vi "NewGame.vi"(7 "GPongType (ChildObject)":refnum<class "GPong.lvclass">, 8 "error in (no error)":errorcluster, 11 "FPGA_ref":T1) -> (0 "error out":errorcluster, 3 "GPong out":refnum<class "GPong.lvclass">)   [LabVIEW 2019, in "RT_Game.lvlib" / "GPong.lvclass"]
uses:
  GPong.lvclass
  C:/Users/FreshBob/Dropbox/VIs/myRIO_GameConsole/RT/RT_Game/Game/Game.lvclass
  FPGA_Interface.ctl
  Game/Game.lvclass/Game.ctl
  GameObject/GameObject.lvclass/GameObject.ctl
  Game/Read Sprite3.vi
  GameObject/Write MinSpeed.vi
  GameObject/Write MaxSpeed.vi
  GameObject/Write MaxSpeedX.vi
  GameObject/Write Damping.vi
  GameObject/Write Gravity.vi
  Game/Write Sprite3.vi
  RT_Sprite/RT_Sprite.lvclass
  C:/Users/FreshBob/Dropbox/VIs/myRIO_GameConsole/RT/RT_Game/GameObject/GameObject.lvclass
  Pong/Pong.lvclass
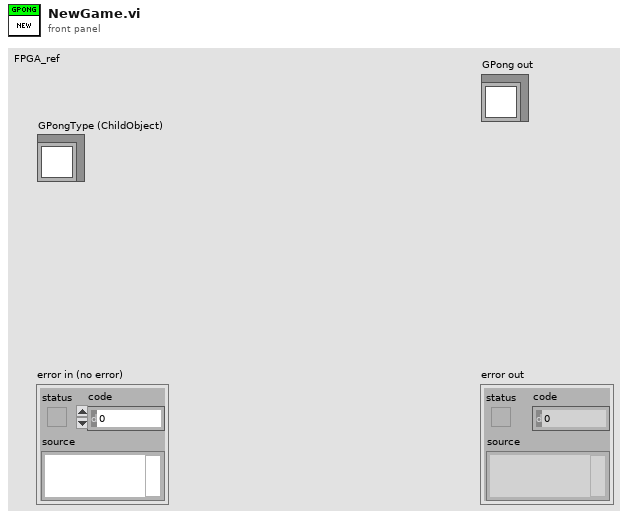
[diagram p1: front panel]
types:
  T1 = typedef "FPGA_Interface.ctl" = refnum<k20>
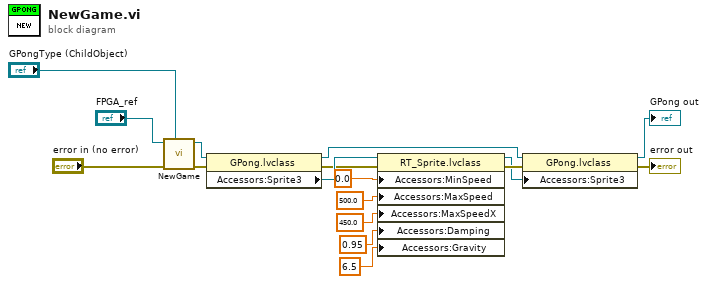
[diagram p0: block diagram]
diagram:
  n1 = call-parent "NewGame.vi"("PongType (ChildObject)"="GPongType (ChildObject)", "error in (no error)"="error in (no error)", "FPGA_ref"="FPGA_ref") -> ("error out"=w17:errorcluster, "Pong out"=w8:refnum<class "GPong.lvclass">)  [unwired: 7 in]
  n2 = property class="GPong.lvclass"(reference=w8, error in=w17) -> (reference out=w3:refnum<class "GPong.lvclass">, error out=w6:errorcluster, "Accessors:Sprite3"=w7:refnum<class "RT_Sprite.lvclass">)
  n3 = property class="RT_Sprite.lvclass"(reference=w7, error in=w6, "Accessors:MinSpeed"=0.0 ("MinSpeed"), "Accessors:MaxSpeed"=500.0 ("MaxSpeed"), "Accessors:MaxSpeedX"=450.0 ("MaxSpeedX"), "Accessors:Damping"=0.95 ("Damping"), "Accessors:Gravity"=6.5 ("Gravity")) -> (reference out=w1:refnum<class "RT_Sprite.lvclass">, error out=w5:errorcluster)
  n4 = property class="GPong.lvclass"(reference=w3, error in=w5, "Accessors:Sprite3"=w1) -> (reference out=→"GPong out":refnum<class "GPong.lvclass">, error out=→"error out":errorcluster)
